vi "AddChildtoNode.vi"(8 "error in":errorcluster, 10 "child in":T1, 11 "CEF_serializable node folder in":refnum<class "CEF_serializable node folder.lvclass">=refnum) -> (0 "error out":errorcluster, 3 "CEF_serializable node folder out":refnum<class "CEF_serializable node folder.lvclass">)   [LabVIEW 2025, in "CEF_serializable node folder.lvclass"]
doc: "Copyright 2017 National Instruments Corporation\n\nLicensed under the Apache License, Version 2.0 (the \"License\"); you may not use this file except in compliance with the License. You may obtain a copy of the License at http://www.apache.org/licenses/LICENSE-2.0\nUnless required by applicable law or agreed to in writing, software distributed under the License is distributed on an \"AS IS\" BASIS, WITHOUT WARRANTIES OR CONDITIONS OF ANY KIND, either express or implied. See the License for the specific language governing permissions and limitations under the License."
uses:
  CEF_serializable node folder.lvclass
  CEF_serializable node folder.lvclass/CEF_serializable node folder.ctl
  <vilib>/NI/Configuration Framework/Node/NISE_CEF_Node.lvclass
  <vilib>/NI/Configuration Framework/Node/NodeRef.ctl
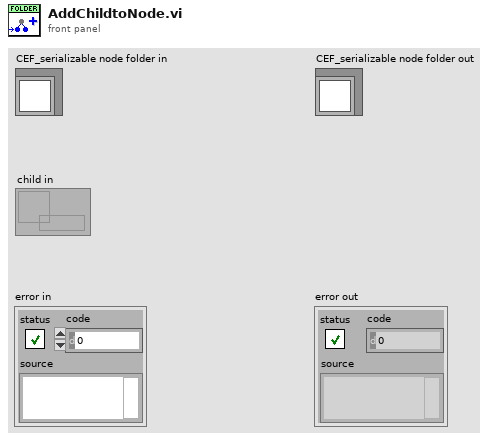
[diagram p1: front panel]
types:
  T1 = typedef "NISE_CEF_Node.lvclass/NodeRef.ctl" = refnum<data-value>
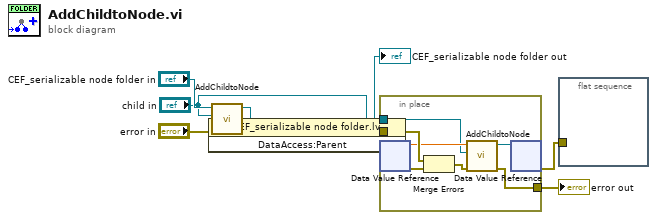
[diagram p0: block diagram]
diagram:
  n1 = call-parent "AddChildtoNode.vi"("error in"="error in", "child in"="child in", "NISE_CEF_Node in"="CEF_serializable node folder in") -> ("error out"=w4:errorcluster, "NISE_CEF_Node out"=w5:refnum<class "CEF_serializable node folder.lvclass">)  [unwired: 7 in]
  n2 = property class="CEF_serializable node folder.lv"(reference=w5, error in=w4) -> (reference out=→"CEF_serializable node folder out":refnum<class "CEF_serializable node folder.lvclass">, error out=w8:errorcluster, "DataAccess:Parent"=w7)
  n3 = in-place {
    in-place-border: w8 -> [w17]
    in-place-border: "child in" -> [w11]
    in-place-border: [w13] -> w1
    n4 = in-place-dvr #1(w7) -> (w15:dbl, w16:errorcluster)
    n5 = Merge Errors(w17, w16) -> (w14:errorcluster)
    n6 = call-dynamic "AddChildtoNode.vi"("error in"=w14, "child in"=w11, "NISE_CEF_Node in"=w15) -> ("error out"=w13:errorcluster, "NISE_CEF_Node out"=w12:refnum<class "NISE_CEF_Node.lvclass">)  [unwired: 7 in]
    n7 = in-place-dvr #1(w12) -> (w6:errorcluster)  [unwired: 1 out]
  }
  "error out" <- w1
  n8 = flat-sequence {
    tunnel: w6 -> [_]
    frame #0 {
    }
  }
